vi "Init Waveform.vi"(8 "error in (no error)":errorcluster, 10 "Units":string, 11 "Tag Name":string) -> (0 "error out":errorcluster, 3 "waveform":waveform(dbl))   [LabVIEW 2023, in "Logger.lvclass"]
uses:
  Logger.lvclass
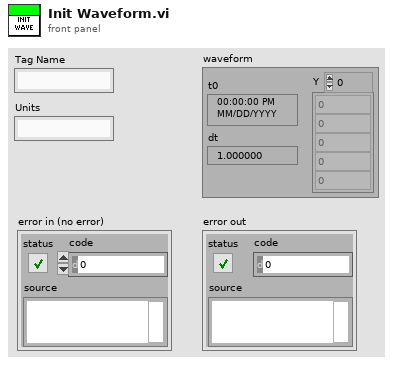
[diagram p1: front panel]
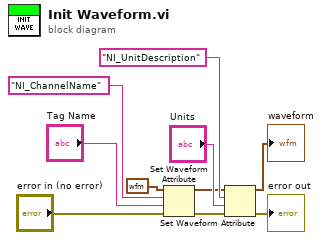
[diagram p0: block diagram]
diagram:
  n1 = Set Waveform Attribute(4:"error in (no error)", 5:"Tag Name", 6:"NI_ChannelName" ("name"), 7:waveform(dbl) {"t0"=timestamp(0 s since 1904-01-01), "dt"=1.0, "Y"=[]} ("waveform")) -> (0:w5:errorcluster, 3:w3:waveform(dbl))  [unwired: 1 out]
  n2 = Set Waveform Attribute(4:w5, 5:"Units", 6:"NI_UnitDescription" ("name"), 7:w3) -> (0:→"error out":errorcluster, 3:→"waveform":waveform(dbl))  [unwired: 1 out]
